vi "Find All Zeros of f(x).vi"   [LabVIEW 2020, in "NI_Gmath.lvlib"]
doc: "Determines all zeros of a 1D function in a given interval. You must manually select the polymorphic instance to use."
uses:
  <vilib>/gmath/NI_Gmath.lvlib
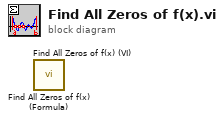
[diagram p0: block diagram]
diagram:
  n1 = call <vilib>:"Find All Zeros of f(x) (Formula).vi"() -> ()  [unwired: 8 in, 4 out]
  n2 = call <vilib>:"Find All Zeros of f(x) (VI).vi"() -> ()  [unwired: 8 in, 4 out]
